vi "gds_tx_send.vi"(8 "error in (no error)":errorcluster, 9 "end of data?":bool, 10 "IQ Data in":cluster{"t0":dbl, "dt":dbl, "Y":cdb[]}={"t0"=0.0, "dt"=1.0, "Y"=[]} {"Y" format="%.3f"; "dt" format="%^.2e"; "t0" format="%.4f"}, 11 "HW parameters in":T1={"Device IP Address"="192.168.11.3", "Active Antenna"="192.168.11.3", "Carrier Frequency (Hz)"=2400000000.0, "Gain (dB)"=2400000000.0, "Generation Mode"=enum."continuous"} {"Gain (dB)" format="%.2f"; "Carrier Frequency (Hz)" format="%.2p"}) -> (0 "error out":errorcluster, 3 "HW parameters out":T1={"Device IP Address"="192.168.11.3", "Active Antenna"="192.168.11.3", "Carrier Frequency (Hz)"=2400000000.0, "Gain (dB)"=2400000000.0, "Generation Mode"=enum."continuous"} {"Gain (dB)" format="%.2f"; "Carrier Frequency (Hz)" format="%.2p"})   [LabVIEW 2012]
uses:
  EE 497/LABS/SDR/control_type_defs.llb/tx_hw params.ctl
  <instrlib>/niUSRP/niUSRP Write Tx Data (CDB Cluster).vi
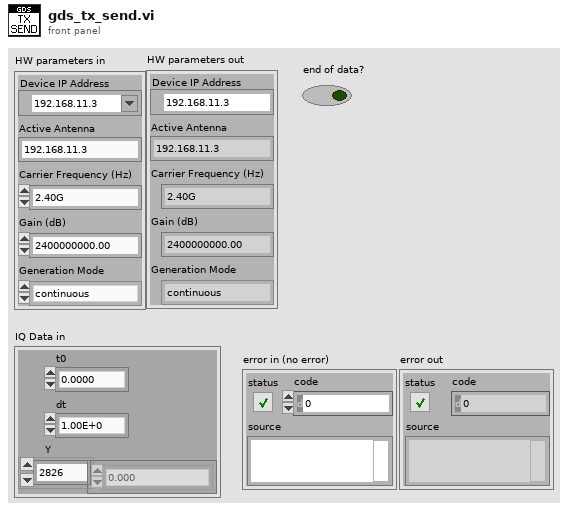
[diagram p1: front panel]
types:
  T1 = typedef "tx_hw params.ctl" = cluster{"Device IP Address":refnum<k15>, "Active Antenna":string, "Carrier Frequency (Hz)":dbl, "Gain (dB)":dbl, "Generation Mode":enum16{"single shot", "simulate", "continuous"}}
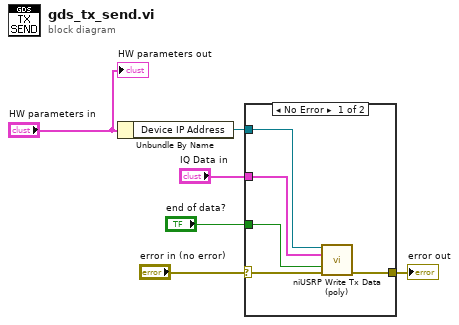
[diagram p0: block diagram]
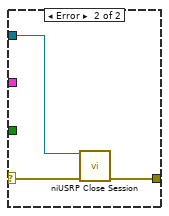
[diagram p2: hidden frame]
diagram:
  n1 = Unbundle By Name("HW parameters in") -> ("Device IP Address"=w3:refnum<k15>)
  n2 = case shown="No Error" "error in (no error)" {
    selector: "error in (no error)" -> [w8 w14]
    tunnel: [w7 w13] -> w5
    tunnel: w3 -> [w11 w12]
    tunnel: "IQ Data in" -> [w10 _]
    tunnel: "end of data?" -> [w9 _]
    frame No Error {
      n3 = call-poly <instrlib>:"niUSRP Write Tx Data (poly).vi"("session handle"=w11, "data"=w10, "end of data?"=w9, "error in (no error)"=w8) -> ("error out"=w7:errorcluster)  [unwired: 10 in, 1 out]
    }
    frame Error {
      n4 = call <instrlib>:"niUSRP Close Session.vi"("session handle"=w12, "error in (no error)"=w14) -> ("error out"=w13:errorcluster)  [unwired: 13 in]
    }
  }
  "error out" <- w5
  "HW parameters out" <- "HW parameters in"
